vi "Done.vi"(8 "error in (no error)":errorcluster, 10 "Philosopher ID":i32, 11 "Table in":refnum<class "Table.lvclass">) -> (0 "error out":errorcluster, 3 "Table out":refnum<class "Table.lvclass">)   [LabVIEW 2023, in "Table.lvlib" / "Table.lvclass"]
uses:
  Table.lvclass
  Fork State.ctl
  Hungry State.ctl
  Table.lvclass/Table.ctl
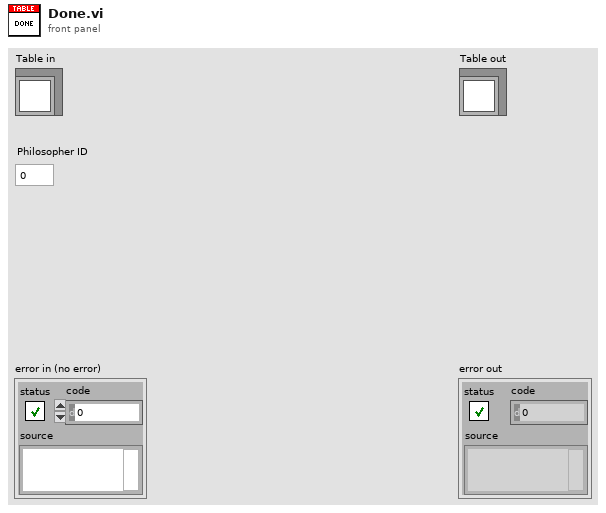
[diagram p1: front panel]
types:
  T1 = typedef "Table.lvlib/Table.lvclass/Hungry State.ctl" = enum16{"NO", "YES"}
  T2 = typedef "Table.lvlib/Table.lvclass/Fork State.ctl" = enum16{"FREE", "IN USE"}
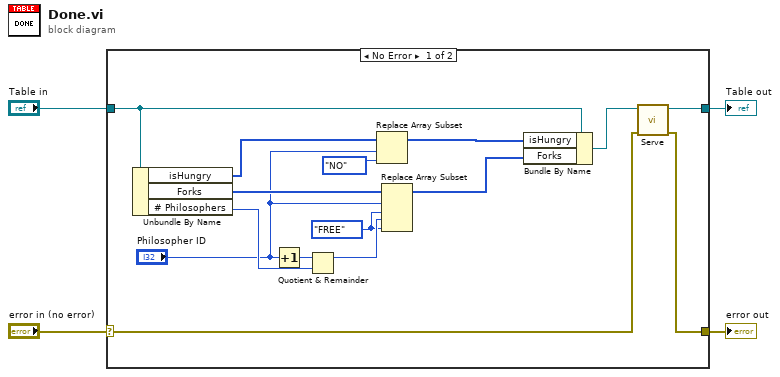
[diagram p0: block diagram]
diagram:
  n1 = case shown="No Error" "error in (no error)" {
    selector: "error in (no error)" -> [w14 w21]
    tunnel: [w13 w21] -> w3
    tunnel: [w15 w20] -> w1
    tunnel: "Table in" -> [w12 w20]
    frame No Error {
      w7 = Fork_State."FREE" ("new element/subarray")
      n2 = Unbundle By Name(w12) -> ("isHungry"=w6:T1[], "Forks"=w19:T2[], "# Philosophers"=w18:i32)
      n3 = Increment(x="Philosopher ID") -> (x+1=w17:i32)
      n4 = Quotient & Remainder(x=w17, y=w18) -> (x-y*floor(x/y)=w9:i32)  [unwired: 1 out]
      n5 = Replace Array Subset(array=w6, new element=Hungry_State."NO" ("new element/subarray"), index="Philosopher ID") -> (w10:T1[])
      n6 = Replace Array Subset(array=w19, new element #1=w7, index #1="Philosopher ID", new element #2=w7, index #2=w9) -> (w8:T2[])
      n7 = Bundle By Name(cluster=w12, "isHungry"=w10, "Forks"=w8) -> (w16:refnum<class "Table.lvclass">)
      n8 = call-dynamic "Serve.vi"("error in (no error)"=w14, "Table in"=w16) -> ("error out"=w13:errorcluster, "Table out"=w15:refnum<class "Table.lvclass">)  [unwired: 8 in]
    }
    frame Error {
    }
  }
  "error out" <- w3
  "Table out" <- w1
